vi "GLdrv_FILE_TRANS_OUTP.vi"(0 "Connection ID":T1, 5 "Start Byte":i32, 7 "End Byte":i32, 11 "error in (no error)":errorcluster, 13 "Query(f)":bool) -> (4 "Connection ID Out":T1, 6 "Data out":string, 15 "error out":errorcluster)   [LabVIEW 2017, in "GL860_Driver.lvlib"]
doc: "記録計本体内のファイルを転送します\nファイルバイト数の設定とデータ転送\nTRANS:OUTP <NR1(転送開始バイト数）>,<NR1(転送終了バイト数)>\n例）　ファイルバイト数が8000バイトの場合\n:FILE:TRANS:OUTP 1,8000 →　：FILE:TRANS:OUTP?\n\nTRANS:OUTP? コマンドの説明\nTRANS:OUTP?を送信すると本体は以下のデータを返します\nヘッダ部：　#6****** (******はヘッダ部、ステータス部を抜いたバイト数の数値が入ります）\nステータス部：　2バイトのバイナリデータ\n1バイト目：　16ビットステータスの上位8ビット\n2バイト目：　16ビットステータスの下位8ビット\n16ビットステータスの内容：　\nビット0：　1=エラーが発生／0=エラーは発生していない\nビット１：　1=転送終了バイト数が不正値／0=OK\nビット２：　1=転送開始バイト数が不正値／0=OK\nデータ部：　ヘッダ部で参照されたバイト数のデータを転送されます\nTRANS 転送コマンドの手順\n１）　:FILE:TRANS:SOUR \"<ファイルパス>”\n２）　:FILE:TRANS:OPEN?\n３）　：FILE:TRANS:SIZE?\n４）　：FILE:TRANS:OUTP <開始バイト>,<終了バイト>\n５）　：FILE：TRANS:OUTP?\n６）　：FILE:TRANS;CLOSE?"
uses:
  GL860_Driver.lvlib
  ConnectionID.ctl
  GLdrv_RW.ctl
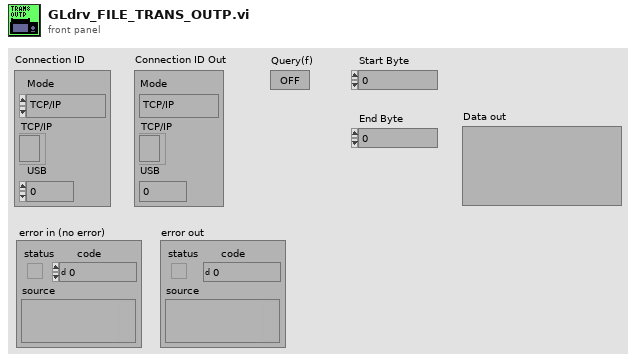
[diagram p1: front panel]
types:
  T1 = typedef "ConnectionID.ctl" = cluster{"Mode":enum16{"TCP/IP", "USB"}, "TCP/IP":refnum<k5>, "USB":i32}
  T2 = typedef "GLdrv_RW.ctl" = enum16{"Auto", "Read", "Write", "Buffer"}
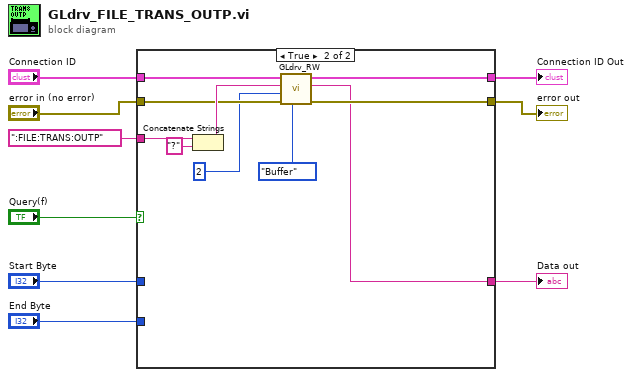
[diagram p0: block diagram]
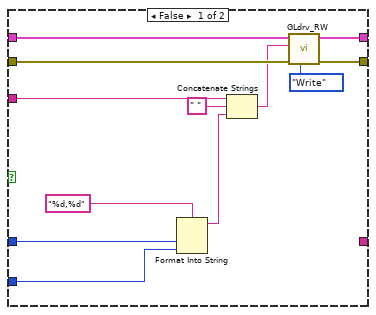
[diagram p2: hidden frame]
diagram:
  n1 = case shown="TRUE" "Query(f)" {
    tunnel: ":FILE:TRANS:OUTP" ("Command") -> [w21 w31]
    tunnel: [w16 w25] -> w9
    tunnel: [w18 w28] -> w8
    tunnel: "Connection ID" -> [w19 w29]
    tunnel: "error in (no error)" -> [w17 w26]
    tunnel: "Start Byte" -> [w12 _]
    tunnel: [_ w23] -> w1
    tunnel: "End Byte" -> [w11 _]
    frame False {
      n2 = Format Into String(format string="%d,%d" ("Param"), w12, w11) -> (resulting string=w13:string)  [unwired: 2 in, 1 out]
      n3 = Concatenate Strings(w21, " " ("string"), w13) -> (w15:string)
      n4 = call "GLdrv_RW.vi"("Mode(read)"=GLdrv_RW."Write", "error in (no error)"=w17, "data in"=w15, "Connection ID"=w19) -> ("error out"=w16:errorcluster, "Connection ID Out"=w18:T1)  [unwired: 3 in, 3 out]
    }
    frame True {
      n5 = Concatenate Strings(w31, "?" ("string")) -> (w27:string)
      n6 = call "GLdrv_RW.vi"("Mode(read)"=GLdrv_RW."Buffer", "error in (no error)"=w26, "Count(0:[CR+LF])"=u32 2, "data in"=w27, "Connection ID"=w29) -> ("error out"=w25:errorcluster, "data out"=w23:string, "Connection ID Out"=w28:T1)  [unwired: 2 in, 2 out]
    }
  }
  "Connection ID Out" <- w8
  "error out" <- w9
  "Data out" <- w1
